vi "DEMO Sequence Execution.vi"() -> (2 "Array":cluster{"AO-64 Array":dbl[], "Command":string}[](array[cluster]), 3 "Repatching steps":T1[](array[typedef]))   [LabVIEW 2018, in "Sequence.lvclass"]
uses:
  Sequence.lvclass
  SequenceSubvis/PatchNewTestStep.ctl
  SequenceSubvis/RF Direction.ctl
  SequenceSubvis/PolarizationSelect.ctl
  APARMainSubvis/VXM Public API/singleAxisMoveDef.ctl
  APARMainSubvis/VXM Public API/mmWaveAxis.ctl
panel:
  in  "Test Type":bool
  out "error out":errorcluster
  in  "Motion Config Park & Measure":bool=TRUE
  out "i":i32=7
  in  "stop":bool
  # "<< off is Patch"
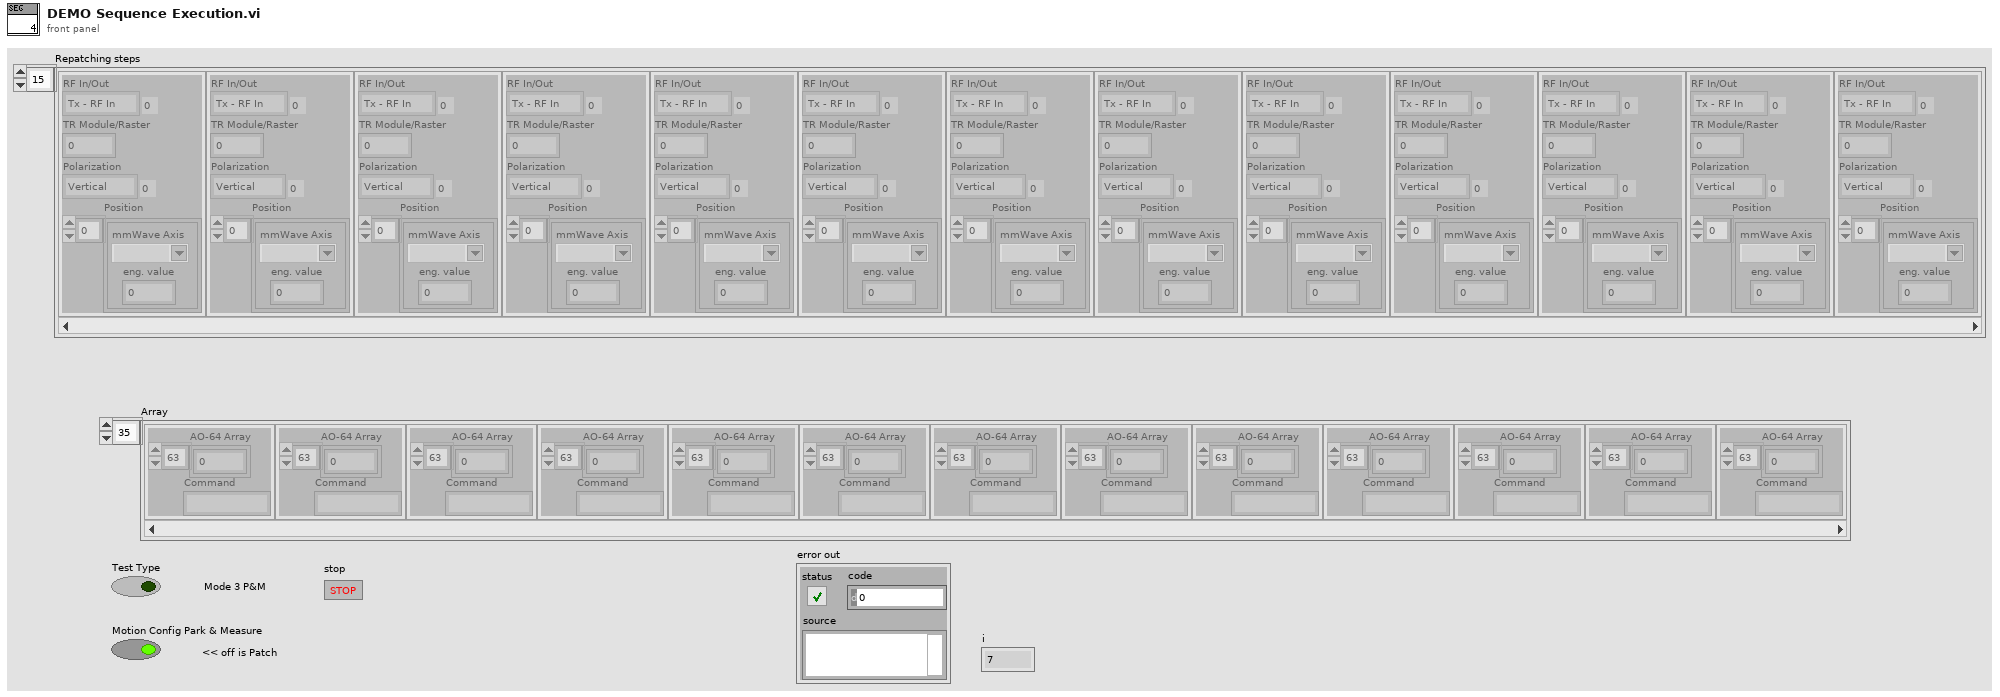
[diagram p1: front panel]
types:
  T1 = typedef "PatchNewTestStep.ctl" = cluster{"RF In/Out":T2, "TR Module/Raster":i32, "Polarization":T3, "Position":T4[]}
  T2 = typedef "RF Direction.ctl" = enum16{"Tx - RF In", "Rx - RF Out"}
  T3 = typedef "PolarizationSelect.ctl" = enum16{"Vertical", "Horizontal"}
  T4 = typedef "singleAxisMoveDef.ctl" = cluster{"mmWave Axis":T5, "eng. value":dbl}
  T5 = typedef "mmWaveAxis.ctl" = string
  T6 = typedef "MultipleMessageQues.ctl" = cluster{"Main que":T7, "Error que":T7, "DAQ que":T7}
  T7 = typedef "MessageQue.lvlib/MessageQue.ctl" = refnum<queue>
  T8 = cluster{path, "Motion Config Park & Measure":bool}
  T9 = typedef "Mode3TestProperties.ctl" = cluster{"Probe Horizontal Polarization":bool, "Probe Vertical Polarization":bool, "Upload TR Module file":path, "Data File Name":string, "RF In/Out of antenna":T2}
  T10 = typedef "mWaveTestStep.ctl" = cluster{"StepType":T11, "RF In/Out":T2, "Module/Raster":i32, "Polarization":T3, "AO-64 Array":dbl[], "Position":T4[]}
  T11 = typedef "TestStepTypes.ctl" = enum16{"MotionFF-M2", "Motion", "SweepTest", "RasterTest", "Finish", "64ModuleCfg"}
  T12 = typedef "Mode1TestProperties.ctl" = cluster{"Probe Horizontal Polarization":bool, "Probe Vertical Polarization":bool, "Data File Name":string, "RF In/Out of antenna":T2, "Raster XY Points":cluster{"X mm":dbl, "Y mm":dbl}[]}
  T13 = typedef "DataLog.lvclass/SearchableTag.ctl" = cluster{"Module, 0-63":i32, "RF Direction Tx0":T2, "Polarization, V0 H1":T3, "AO-64 Array":dbl[]}
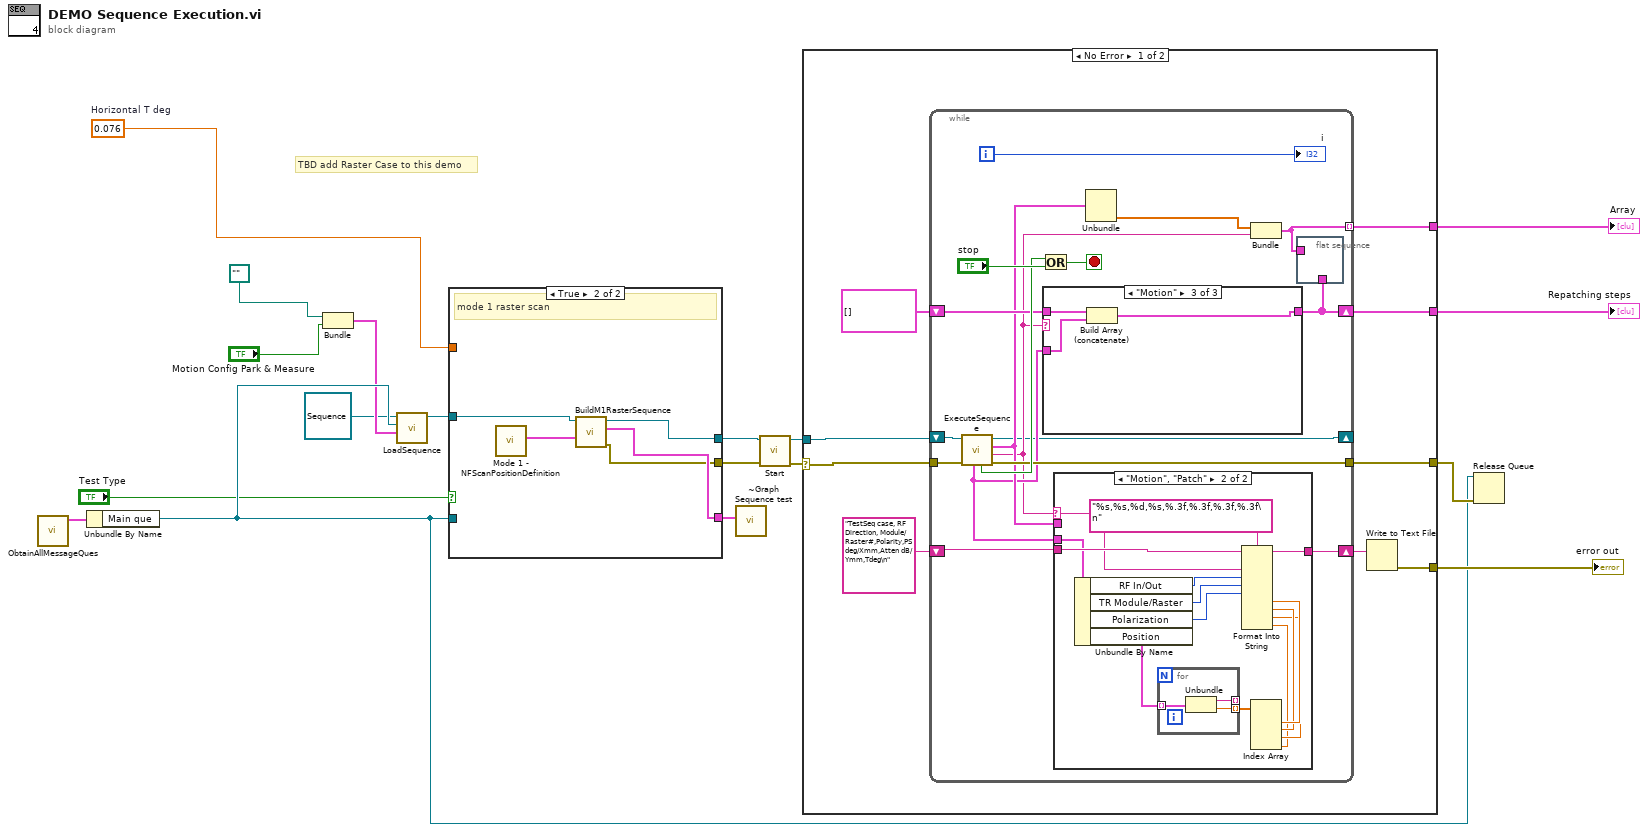
[diagram p0: block diagram]
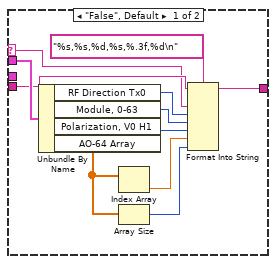
[diagram p2: hidden frame]
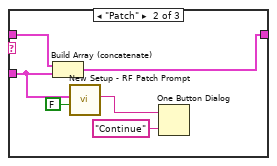
[diagram p4: hidden frame]
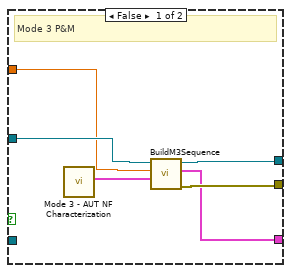
[diagram p6: hidden frame]
diagram:
  w1 = 0.076  # Horizontal T deg
  # "TBD add Raster Case to this demo"
  n1 = call "ObtainAllMessageQues.vi"() -> ("MessageQues"=w10:T6)  [unwired: 10 in, 1 out]
  n2 = Unbundle By Name(w10) -> ("Main que"=w9:T7)
  n3 = Bundle(path "", "Motion Config Park & Measure"="Motion Config Park & Measure") -> (w6:T8)  [unwired: 1 in]
  n4 = call "LoadSequence.vi"("Sequence Cfg"=w6, "Message que"=w9, "Sequence in"=refnum<class "Sequence.lvclass"> refnum) -> ("Sequence out"=w4:refnum<class "Sequence.lvclass">)  [unwired: 7 in, 1 out]
  n5 = case shown="True" "Test Type" {
    tunnel: [w23 w27] -> w16
    tunnel: [w22 w25] -> w14
    tunnel: [w19 w26] -> w12
    tunnel: w9 -> [_ _]
    tunnel: w4 -> [w21 w28]
    tunnel: w1 -> [w20 _]
    frame False {
      # "Mode 3 P&M"
      n6 = call "Mode 3 - AUT NF Characterization.vi"() -> ("Mode3 Test Properties"=w24:T9)  [unwired: 10 in, 1 out]
      n7 = call "BuildM3Sequence.vi"("Mode3 Test Properties"=w24, "Horizontal T deg"=w20, "Sequence in"=w21) -> ("error out"=w22:errorcluster, "PAARD Test Sequence"=w19:T10[], "Sequence out"=w23:refnum<class "Sequence.lvclass">)  [unwired: 5 in, 1 out]
    }
    frame True {
      # "mode 1 raster scan"
      n8 = call "Mode 1 - NFScanPositionDefinition.vi"() -> ("Mode3TestProperties"=w29:T12)  [unwired: 10 in, 1 out]
      n9 = call "BuildM1RasterSequence.vi"("Mode3TestProperties"=w29, "Sequence in"=w28) -> ("error out"=w25:errorcluster, "PAARD Test Sequence"=w26:T10[], "Sequence out"=w27:refnum<class "Sequence.lvclass">)  [unwired: 6 in, 1 out]
    }
  }
  n10 = call "~Graph Sequence test.vi"("PAARD Test Seq"=w12) -> ()  [unwired: 11 in]
  n11 = call "Start.vi"("error in (no error)"=w14, "Sequence in"=w16) -> ("error out"=w3:errorcluster, "Sequence out"=w15:refnum<class "Sequence.lvclass">)  [unwired: 8 in]
  n12 = case shown="No Error" w3 {
    selector: w3 -> [w33 w94]
    tunnel: [w38 _] -> w18
    tunnel: [w37 _] -> w17
    tunnel: w15 -> [w36 _]
    tunnel: [w35 _] -> w13
    tunnel: [w34 w94] -> w11
    frame No Error {
      n13 = while {
        tunnel: w33 -> [w52]
        tunnel: [w47] -> w38 mode=indexing
        shift-right: [w46] -> w37
        shift-left: T1[] [] -> [w51]
        shift-right: [w40] -> _
        shift-left: w36 -> [w49]
        tunnel: [w48] -> w35
        shift-right: [w41] -> w31
        shift-left: "TestSeq case, RF Direction, Module/Raster#,Polarity,PS deg/Xmm,Atten dB/Ymm,Tdeg\n" -> [w42]
        i -> [w50]
        stop <- w53 stop-if-true
        n14 = call "ExecuteSequence.vi"("error in (no error)"=w52, "Sequence in"=w49) -> ("error out"=w48:errorcluster, "Command"=w43:string, "SweepProperties"=w45:T13, "Sequence out"=w40:refnum<class "Sequence.lvclass">, "Sequence is done"=w54:bool, "Next Position"=w44:T1)  [unwired: 4 in]
        n15 = Or(x=w54, y="stop") -> (x .or. y?=w53:bool)
        n16 = case shown="\"Motion\"" w43 {
          tunnel: w51 -> [w84 w90 w93]
          tunnel: w44 -> [_ w88 w91]
          tunnel: [w84 w89 w92] -> w46
          frame "False", Default {
          }
          frame "Patch" {
            n17 = Build Array (concatenate)(w90, w88) -> (w89:T1[])
            n18 = call "New Setup - RF Patch Prompt.vi"("Motion"=FALSE, "NewSetup"=w88) -> ("Dialog Prompt"=w87:string)  [unwired: 9 in]
            n19 = One Button Dialog(message=w87, button name ("OK")="Continue") -> ()  [unwired: 1 out]
          }
          frame "Motion" {
            n20 = Build Array (concatenate)(w93, w91) -> (w92:T1[])
          }
        }
        n21 = case shown="\"Motion\", \"Patch\"" w43 {
          selector: w43 -> [w60 w76]
          tunnel: w45 -> [w65 _]
          tunnel: w44 -> [_ w78]
          tunnel: w42 -> [w63 w79]
          tunnel: [w64 w77] -> w41
          frame "False", Default {
            n22 = Unbundle By Name(w65) -> ("RF Direction Tx0"=w62:T2, "Module, 0-63"=w59:i32, "Polarization, V0 H1"=w61:T3, "AO-64 Array"=w58:dbl[])
            n23 = Index Array(array=w58) -> (element=w57:dbl)  [unwired: 1 in]
            n24 = Array Size(array=w58) -> (size(s)=w56:i32)
            n25 = Format Into String(format string="%s,%s,%d,%s,%.3f,%d\n", initial string=w63, w60, w62, w59, w61, w57, w56) -> (resulting string=w64:string)  [unwired: 1 in, 1 out]
          }
          frame "Motion", "Patch" {
            n26 = Unbundle By Name(w78) -> ("RF In/Out"=w75:T2, "TR Module/Raster"=w74:i32, "Polarization"=w73:T3, "Position"=w72:T4[])
            n27 = for {
              tunnel: w72 -> [w83] mode=indexing
              tunnel: [w82] -> _ mode=indexing
              tunnel: [w81] -> w71 mode=indexing
              n28 = Unbundle(w83) -> ("mmWave Axis"=w82:T5, "eng. value"=w81:dbl)
            }
            n29 = Index Array(array=w71) -> (element #1=w70:dbl, element #2=w69:dbl, element #3=w68:dbl, element #4=w67:dbl)  [unwired: 4 in]
            n30 = Format Into String(format string="%s,%s,%d,%s,%.3f,%.3f,%.3f,%.3f\n", initial string=w79, w76, w75, w74, w73, w70, w69, w68, w67) -> (resulting string=w77:string)  [unwired: 1 in, 1 out]
          }
        }
        n31 = Unbundle(w45) -> ("AO-64 Array"=w39:dbl[])  [unwired: 3 out]
        n32 = Bundle("AO-64 Array"=w39, "Command"=w43) -> (w47:cluster{"AO-64 Array":dbl[], "Command":string})  [unwired: 1 in]
        n33 = flat-sequence {
          tunnel: w47 -> [_]
          tunnel: w46 -> [_]
          frame #0 {
          }
        }
        "i" <- w50
      }
      n34 = Write to Text File(text=w31) -> (error out=w34:errorcluster)  [unwired: 3 in, 2 out]
    }
    frame Error {
    }
  }
  "Array" <- w18
  "Repatching steps" <- w17
  "error out" <- w11
  n35 = Release Queue(queue=w9, error in (no error)=w13) -> ()  [unwired: 1 in, 3 out]
